vi "导出差值数据.vi"(8 "error in":errorcluster, 9 "COM":i32=4, 10 "阀值":dbl, 11 "IN":i32=129) -> (0 "error out":errorcluster)   [LabVIEW 2015]
uses:
  <vilib>/Utility/NIReport.llb/NI_report.lvclass
  <vilib>/Utility/NIReport.llb/Excel/NI_Excel.lvclass
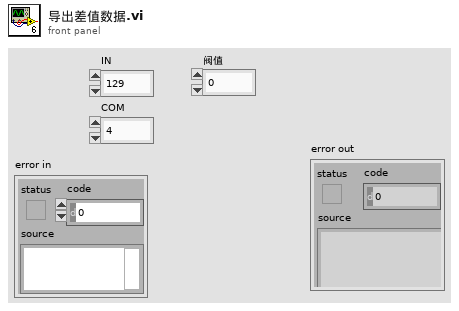
[diagram p1: front panel]
types:
  T1 = enum16{"Standard Report", "HTML", "Word", "Excel"}
  T2 = enum16{"maximized", "minimized", "normal", "no change"}
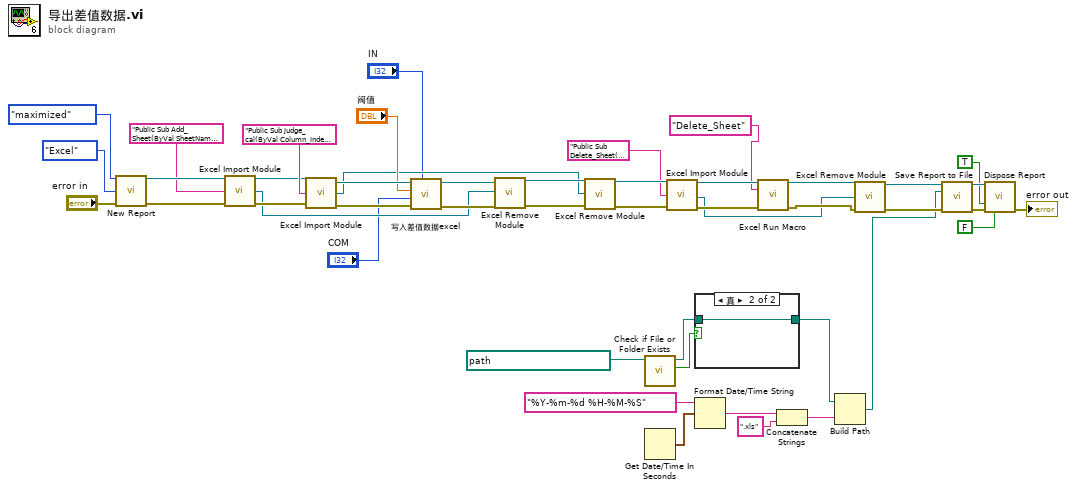
[diagram p0: block diagram]
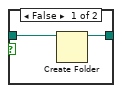
[diagram p2: hidden frame]
diagram:
  n1 = call <vilib>:"New Report.vi"("window state (normal)"=T2."maximized", "report type"=T1."Excel", "error in (no error)"="error in") -> ("report out"=w43:refnum<class "NI_report.lvclass">, "error out"=w42:errorcluster)  [unwired: 11 in]
  n2 = call <vilib>:"Excel Import Module.vi"("report in"=w43, "module code (\"\")"="Public Sub Add_Sheet(ByVal SheetName As String)\n    Dim shcount As Integer\n    shcount = Sheets.Count\n    Sheets.Add after:=Sheets(shcount)\n    shcount = shcount + 1\n    Sheets(shcount).Name = SheetName\nEnd Sub" ("module code (\"\")"), "error in (no error)"=w42) -> ("report out"=w38:refnum<class "NI_report.lvclass">, "module reference"=w30:refnum<k7>, "error out"=w39:errorcluster)  [unwired: 10 in]
  n3 = call <vilib>:"Excel Import Module.vi"("report in"=w38, "module code (\"\")"="Public Sub judge_cal(ByVal Column_Index As Single, ByVal limit As Single)\n    Dim iRows, i As Integer\n    Dim formu As String\n    Dim loc As Range\n    Dim letter As String\n    iRows = ActiveSheet.UsedRange.Rows.Count\n    For i = 2 To iRows\n        letter = VBA.Split(Cells(1, Column_Index).Address, \"$\")(1)\n        Set loc = Range(letter & i)\n        If abs(loc.Value) > limit Then\n            loc.Font.Color = -16776961\n        End If\n    Next\nEnd Sub" ("module code (\"\")"), "error in (no error)"=w39) -> ("report out"=w37:refnum<class "NI_report.lvclass">, "module reference"=w29:refnum<k7>, "error out"=w36:errorcluster)  [unwired: 10 in]
  n4 = call "写入差值数据excel.vi"("IN"="IN", "error in (no error)"=w36, "COM"="COM", "差值限"="阀值", "NI_report in"=w37) -> ("error out"=w33:errorcluster, "NI_report out"=w34:refnum<class "NI_report.lvclass">)  [unwired: 5 in]
  n5 = call <vilib>:"Excel Remove Module.vi"("report in"=w34, "module reference"=w30, "error in (no error)"=w33) -> ("report out"=w32:refnum<class "NI_report.lvclass">, "error out"=w31:errorcluster)  [unwired: 11 in]
  n6 = call <vilib>:"Excel Remove Module.vi"("report in"=w32, "module reference"=w29, "error in (no error)"=w31) -> ("report out"=w28:refnum<class "NI_report.lvclass">, "error out"=w27:errorcluster)  [unwired: 11 in]
  n7 = call <vilib>:"Check if File or Folder Exists.vi"("path"=path "D:/128X4数据/差值数据" ("base path")) -> ("file or folder exists?"=w10:bool, "dup path"=w11:path)  [unwired: 8 in, 1 out]
  n8 = Get Date/Time In Seconds() -> (seconds since 1Jan1904=w8:timestamp)
  n9 = call <vilib>:"Excel Import Module.vi"("report in"=w28, "module code (\"\")"="Public Sub Delete_Sheet()\n    Application.DisplayAlerts = False\nSheets(\"Sheet1\").Delete\n    Sheets(\"Sheet2\").Delete\n    Sheets(\"Sheet3\").Delete\n    Application.DisplayAlerts = True\nEnd Sub" ("module code (\"\")"), "error in (no error)"=w27) -> ("report out"=w25:refnum<class "NI_report.lvclass">, "module reference"=w20:refnum<k7>, "error out"=w24:errorcluster)  [unwired: 10 in]
  n10 = case shown="真" w10 {
    tunnel: w11 -> [w48 w49]
    tunnel: [w47 w49] -> w12
    frame False {
      n11 = Create Folder(path (use dialog)=w48) -> (created path=w47:path)  [unwired: 2 in, 2 out]
    }
    frame True {
    }
  }
  n12 = Format Date/Time String(time format string (%c)="%Y-%m-%d %H-%M-%S", seconds (now)=w8) -> (date/time string=w5:string)  [unwired: 1 in]
  n13 = call <vilib>:"Excel Run Macro.vi"("report in"=w25, "macro name"="Delete_Sheet", "error in (no error)"=w24) -> ("report out"=w22:refnum<class "NI_report.lvclass">, "error out"=w21:errorcluster)  [unwired: 10 in, 1 out]
  n14 = Concatenate Strings(w5, ".xls") -> (w4:string)
  n15 = Build Path(base path=w12, name or relative path=w4) -> (appended path=w3:path)
  n16 = call <vilib>:"Excel Remove Module.vi"("report in"=w22, "module reference"=w20, "error in (no error)"=w21) -> ("report out"=w14:refnum<class "NI_report.lvclass">, "error out"=w13:errorcluster)  [unwired: 11 in]
  n17 = call-dynamic "Save Report to File.vi"("report in"=w14, "report file path"=w3, "error in (no error)"=w13) -> ("report out"=w19:refnum<class "NI_report.lvclass">, "error out"=w18:errorcluster)  [unwired: 11 in]
  n18 = call-dynamic "Dispose Report.vi"("report in"=w19, "save changes? (F)"=TRUE, "error in (no error)"=w18, "close report? (T)"=FALSE) -> ("error out"=→"error out":errorcluster)  [unwired: 11 in]
